vi "FacadeResizable1DArray(String).vi"(0 "Data In":T4, 2 "Display State In":T2, 3 "Container State":T3) -> (6 "Data Out":T4, 7 "Display State Out":T2, 8 "Action":T1)   [LabVIEW 2011, in "Resizable1DArray(String).xctl"]
uses:
  <vilib>/_probes/SAPHIR/ViBox - Probes/Resizable1DArray/Resizable1DArray(String)/Resizable1DArray(String).xctl
  <vilib>/_probes/SAPHIR/ViBox - Probes/Resizable1DArray/Resizable1DArray(String)/DataResizable1DArray(String).ctl
  <vilib>/_xctls/Container State.ctl
  <vilib>/_probes/SAPHIR/ViBox - Probes/Resizable1DArray/Resizable1DArray(String)/StateResizable1DArray(String).ctl
  <vilib>/_xctls/Action.ctl
  <vilib>/_xctls/XControlSupport.lvlib
panel:
  out "String":string
  in  "DisplayFormat":enum16{"Normal", "Code", "Hex"}(ring) caption="Display format :"
  out "[Strings]":string[](array[string])
  # "Display Options"
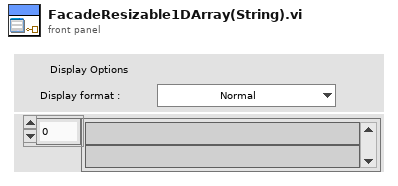
[diagram p1: front panel]
types:
  T1 = typedef "XControlSupport.lvlib/Action.ctl" = cluster{"Data Changed?":bool, "State Changed?":bool, "Action Name":string}
  T2 = typedef "Resizable1DArray(String).xctl/StateResizable1DArray(String).ctl" = cluster{"Height":u32}
  T3 = typedef "XControlSupport.lvlib/Container State.ctl" = cluster{"Indicator?":bool, "Run Mode?":bool, " Refnum":refnum<vi>}
  T4 = typedef "Resizable1DArray(String).xctl/DataResizable1DArray(String).ctl" = string[]
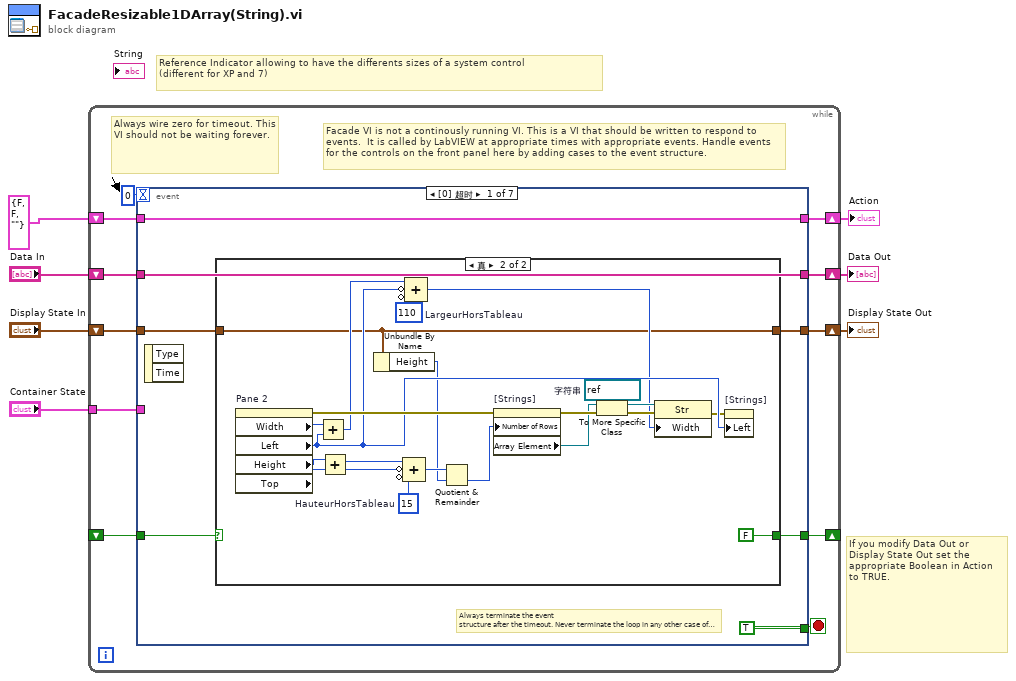
[diagram p0: block diagram]
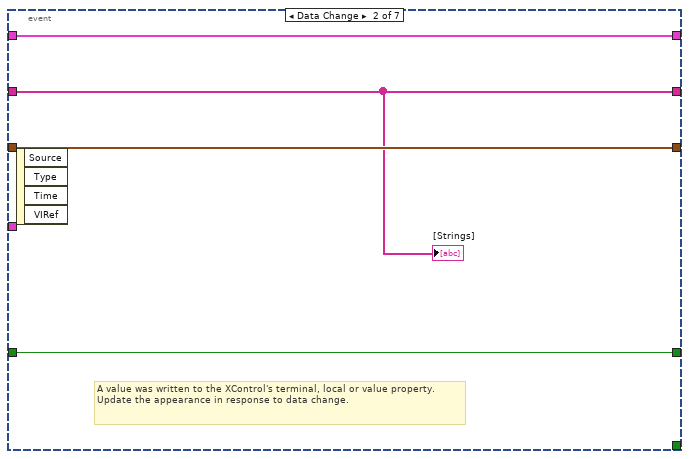
[diagram p3: hidden frame]
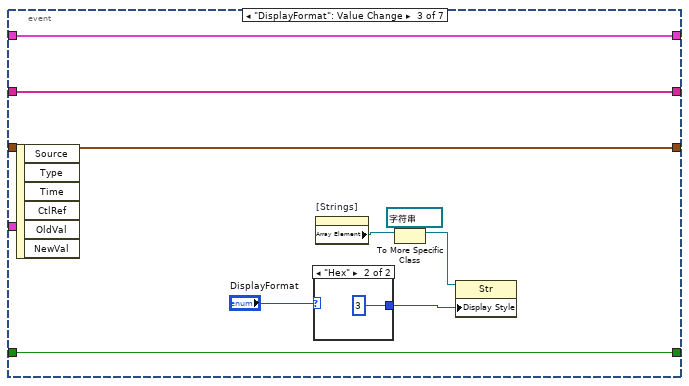
[diagram p4: hidden frame]
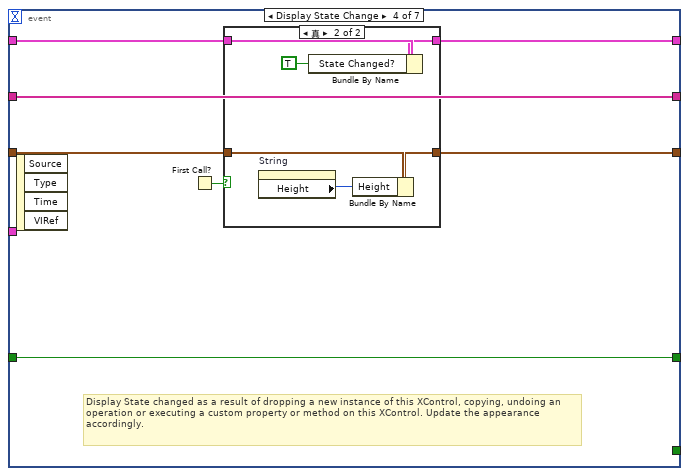
[diagram p6: hidden frame]
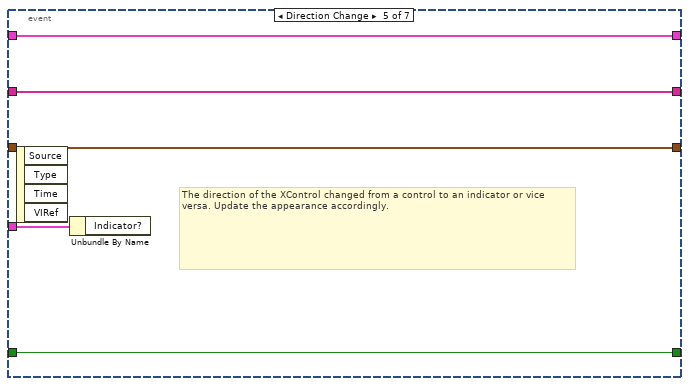
[diagram p8: hidden frame]
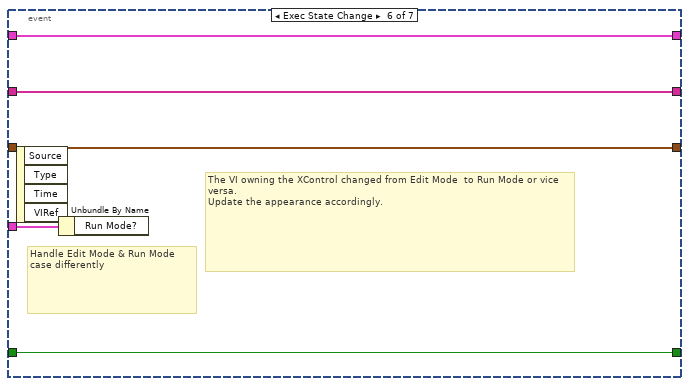
[diagram p9: hidden frame]
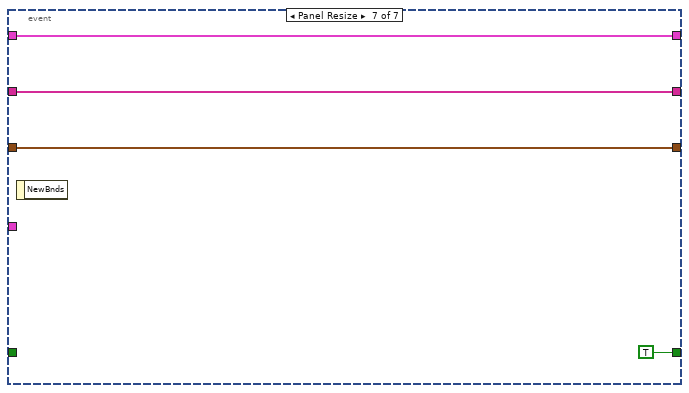
[diagram p10: hidden frame]
diagram:
  # "Reference Indicator allowing to have the differents sizes of a system control\n(different for XP and 7)"
  # "If you modify Data Out or\nDisplay State Out set the\nappropriate Boolean in Action\nto TRUE."
  n1 = while {
    shift-right: [w17] -> w5
    shift-left: "Display State In" -> [w18]
    tunnel: "Container State" -> [w14]
    shift-right: [w12] -> w7
    shift-left: "Data In" -> [w13]
    shift-right: [w10] -> w3
    shift-left: T1 {"Data Changed?"=FALSE, "State Changed?"=FALSE, "Action Name"=""} ("Action") -> [w11]
    shift-right: [w8] -> _
    shift-left: _ -> [w9]
    stop <- w16 stop-if-true
    # "Facade VI is not a continously running VI. This is a VI that should be written to respond to events.  It is called by LabVIEW at appropriate times with appropriate events. Handle events for the controls on the front panel here by adding cases to the event structure."
    # "Always wire zero for timeout. This\nVI should not be waiting forever."
    n2 = event shown="[0] 超时" {
      selector: _ -> [_ _ _ _ _ _ _]
      dyn-events: _ -> [_ _ _ _ _ _ _]
      timeout: 0 -> [_ _ _ _ _ _ _]
      tunnel: w18 -> [w20 w52 w56 w67 w82 w87 w91]
      tunnel: [w19 w52 w56 w66 w82 w87 w91] -> w17
      tunnel: [TRUE _ _ _ _ _ _] -> w16
      tunnel: w14 -> [_ _ _ _ w83 w88 _]
      tunnel: w13 -> [w23 w50 w55 w70 w81 w86 w92]
      tunnel: [w23 w50 w55 w70 w81 w86 w92] -> w12
      tunnel: [w24 w51 w54 w64 w80 w85 w90] -> w10
      tunnel: w11 -> [w24 w51 w54 w65 w80 w85 w90]
      tunnel: w9 -> [w22 w49 w53 w69 w79 w84 _]
      tunnel: [w21 w49 w53 w69 w79 w84 TRUE] -> w8
      event Timeout {
        # "Always terminate the event\nstructure after the timeout. Never terminate the loop in any other case of the event structure."
        n3 = event-data() -> ()  [unwired: 3 out]
        n4 = case shown="真" w22 {
          selector: w22 -> [w27 _]
          tunnel: [w27 FALSE] -> w21
          tunnel: w20 -> [w26 w30]
          tunnel: [w26 w30] -> w19
          frame False {
          }
          frame True {
            w35 = refnum<vi> refnum  # 字符串
            w33 = i16 15  # HauteurHorsTableau
            w34 = i16 110  # LargeurHorsTableau
            n5 = property on="Pane 2" class="Pane"() -> (error out=w46:errorcluster, "Width"=w44:u32, "Left"=w43:i32, "Height"=w48:u32, "Top"=w47:i32)  [unwired: 2 in, 1 out]
            n6 = Add(x=w44, y=w43) -> (x+y=w42:u32)
            n7 = Add(x=w48, y=w47) -> (x+y=w45:u32)
            n8 = Unbundle By Name(w30) -> ("Height"=w29:u32)
            n9 = Compound Arithmetic op=ADD(w45, invert w47, invert w33) -> (w38:u32)
            n10 = Compound Arithmetic op=ADD(w42, invert w43, invert w34) -> (w32:u32)
            n11 = Quotient & Remainder(x=w38, y=w29) -> (floor(x/y)=w28:u32)  [unwired: 1 out]
            n12 = property on="[Strings]" class="Arr (严格)"(error in=w46, "Number of Rows"=w28) -> (error out=w39:errorcluster, "Array Element"=w37:refnum<vi>)  [unwired: 1 in, 1 out]
            n13 = To More Specific Class(target class=w35, reference=w37, error in=w39) -> (specific class reference=w36:refnum<vi>, error out=w40:errorcluster)
            n14 = property class="Str"(reference=w36, error in=w40, "Width"=w32) -> (error out=w41:errorcluster)  [unwired: 1 out]
            n15 = property on="[Strings]" class="Arr (严格)"(error in=w41, "Left"=w43) -> ()  [unwired: 1 in, 2 out]
          }
        }
      }
      event Data Change {
        # "A value was written to the XControl's terminal, local or value property.\nUpdate the appearance in response to data change."
        n16 = event-data() -> ()  [unwired: 5 out]
        "[Strings]" <- w50
      }
      event "DisplayFormat": Value Change {
        n17 = event-data() -> ()  [unwired: 7 out]
        n18 = case shown="\"Hex\"" "DisplayFormat" {
          selector: "DisplayFormat" -> [w62 _]
          tunnel: [w62 u32 3 ("Display Style")] -> w58
          frame Default {
          }
          frame "Hex" {
          }
        }
        n19 = property on="[Strings]" class="Arr (严格)"() -> ("Array Element"=w61:refnum<vi>)  [unwired: 2 in, 2 out]
        n20 = To More Specific Class(target class=refnum<vi> refnum ("specific class reference"), reference=w61) -> (specific class reference=w59:refnum<vi>)  [unwired: 1 in, 1 out]
        n21 = property class="Str"(reference=w59, "Display Style"=w58) -> ()  [unwired: 1 in, 2 out]
      }
      event Display State Change {
        # "Display State changed as a result of dropping a new instance of this XControl, copying, undoing an operation or executing a custom property or method on this XControl. Update the appearance accordingly."
        n22 = event-data() -> ()  [unwired: 5 out]
        n23 = First Call?() -> (First Call?: T/F=w68:bool)
        n24 = case shown="真" w68 {
          tunnel: w67 -> [w72 w78]
          tunnel: [w72 w77] -> w66
          tunnel: w65 -> [w71 w75]
          tunnel: [w71 w74] -> w64
          frame False {
          }
          frame True {
            n25 = property on="String" class="Str"() -> ("Height"=w76:u32)  [unwired: 2 in, 2 out]
            n26 = Bundle By Name(cluster=w75, "State Changed?"=TRUE) -> (w74:T1)
            n27 = Bundle By Name(cluster=w78, "Height"=w76) -> (w77:T2)
          }
        }
      }
      event Direction Change {
        # "The direction of the XControl changed from a control to an indicator or vice versa. Update the appearance accordingly."
        n28 = event-data() -> ()  [unwired: 5 out]
        n29 = Unbundle By Name(w83) -> ()  [unwired: 1 out]
      }
      event Exec State Change {
        # "The VI owning the XControl changed from Edit Mode  to Run Mode or vice versa.\nUpdate the appearance accordingly."
        # "Handle Edit Mode & Run Mode\ncase differently"
        n30 = event-data() -> ()  [unwired: 5 out]
        n31 = Unbundle By Name(w88) -> ()  [unwired: 1 out]
      }
      event Panel Resize {
        n32 = event-data() -> ()  [unwired: 2 out]
      }
    }
  }
  "Display State Out" <- w5
  "Data Out" <- w7
  "Action" <- w3
